vi "FlipColor.vi"(10 "Current Color":u32(colorbox), 11 "BarCode in":refnum<class "BarCode.lvclass">) -> (2 "Next color":u32(colorbox), 3 "BarCode out":refnum<class "BarCode.lvclass">)   [LabVIEW 2013, in "BarCodes.lvlib" / "BarCode.lvclass"]
uses:
  BarCode.lvclass
  Read Dark Color.vi
  Read Light Color.vi
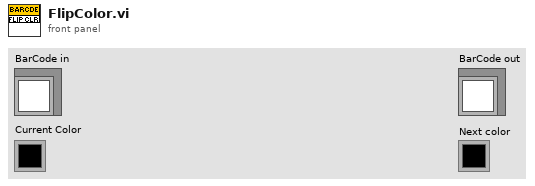
[diagram p1: front panel]
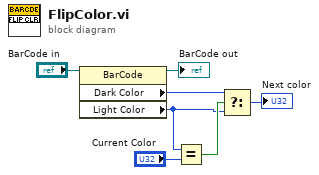
[diagram p0: block diagram]
diagram:
  n1 = property class="BarCode"(reference="BarCode in") -> (reference out=→"BarCode out":refnum<class "BarCode.lvclass">, "Dark Color"=w5:u32, "Light Color"=w4:u32)  [unwired: 1 in, 1 out]
  n2 = Equal?(x=w4, y="Current Color") -> (x = y?=w6:bool)
  n3 = Select(t=w5, s=w6, f=w4) -> (s? t:f=→"Next color":u32)
